vi "push array poli.vi"   [LabVIEW 2010, in "Licor-Steuerung.lvlib"]
uses:
  Licor-Steuerung.lvlib
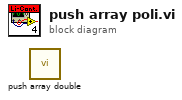
[diagram p0: block diagram]
diagram:
  n1 = call "push array double.vi"() -> ()  [unwired: 15 in, 1 out]
